vi "Func_ChangeControl.vi"(8 "error in (no error)":errorcluster, 10 "Control Path":path, 11 "Control in":refnum<vi>) -> (0 "error out":errorcluster, 3 "GObject out":refnum<vi>)   [LabVIEW 2010, in "TemplateGenerator.lvlib"]
uses:
  TemplateGenerator.lvlib
  <vilib>/Utility/miscctls.llb/LVPointTypeDef.ctl
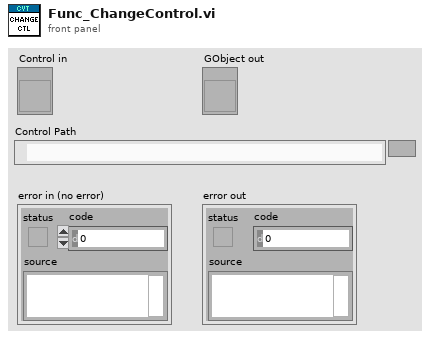
[diagram p1: front panel]
types:
  T1 = typedef "LVPointTypeDef.ctl" = cluster{"Horizontal":i16, "Vertical":i16}
  T2 = typedef "LVNumericRepresentation.ctl" = enum32{"Extended Precision", "Double Precision", "Single Precision", "Long", "Word", "Byte", "Unsigned Long", "Unsigned Word", "Unsigned Byte", "Complex Extended", "Complex Double", "Complex Single", "Quad", "Unsigned Quad", "Fixed-Point"}
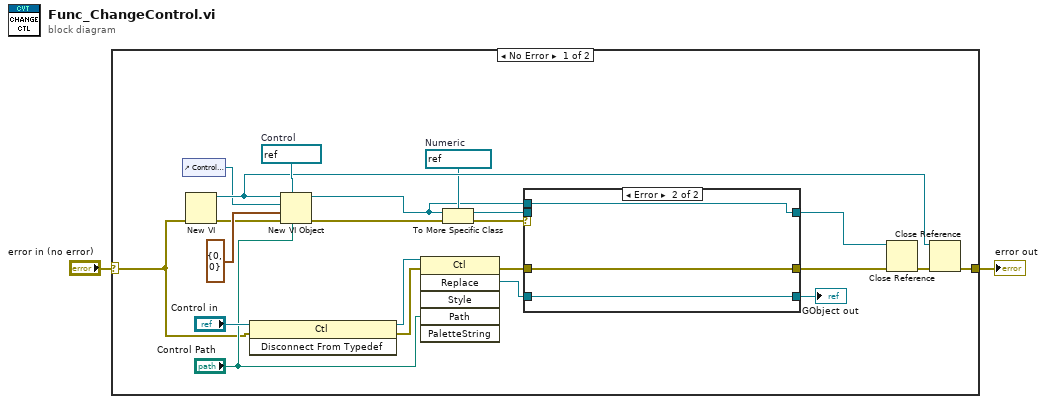
[diagram p0: block diagram]
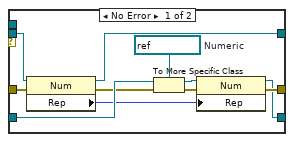
[diagram p2: hidden frame]
diagram:
  n1 = case shown="No Error" "error in (no error)" {
    selector: "error in (no error)" -> [w4 w39]
    tunnel: [w6 w39] -> w2
    frame No Error {
      w17 = refnum<vi> refnum  # Numeric
      w21 = refnum<vi> refnum  # Control
      n2 = control-ref of="Control Path"() -> (w15:refnum<vi>)
      n3 = New VI(8:w4) -> (0:w18:errorcluster, 3:w19:refnum<vi>)  [unwired: 6 in]
      n4 = invoke class="Ctl" method="Disconnect From Typedef"(reference="Control in", error in=w4) -> (reference out=w23:refnum<vi>, error out=w24:errorcluster)  [unwired: 1 in, 1 out]
      n5 = New VI Object(vi object class=w21, owner refnum=w19, style=w15, position/next to=T1 {"Horizontal"=0, "Vertical"=0} ("location"), 6:"Control Path", 8:w18) -> (object refnum=w3:refnum<vi>, 0:w10:errorcluster)  [unwired: 2 in]
      n6 = invoke class="Ctl" method="Replace"(reference=w23, error in=w24, "Path"="Control Path") -> (error out=w5:errorcluster, "Replace"=w13:refnum<vi>)  [unwired: 3 in, 4 out]
      n7 = To More Specific Class(target class=w17, reference=w3, error in=w10) -> (specific class reference=w12:refnum<vi>, error out=w14:errorcluster)
      n8 = case shown="Error" w14 {
        tunnel: w13 -> [w32 w38]
        tunnel: w5 -> [w35 w37]
        tunnel: w12 -> [w34 _]
        tunnel: [w33 w36] -> w11
        tunnel: [w26 w37] -> w8
        tunnel: [w25 w38] -> w9
        tunnel: w3 -> [_ w36]
        frame No Error {
          w31 = refnum<vi> refnum  # Numeric
          n9 = property class="Num"(reference=w34, error in=w35) -> (reference out=w33:refnum<vi>, error out=w29:errorcluster, "Rep"=w27:T2)
          n10 = To More Specific Class(target class=w31, reference=w32, error in=w29) -> (specific class reference=w30:refnum<vi>, error out=w28:errorcluster)
          n11 = property class="Num"(reference=w30, error in=w28, "Rep"=w27) -> (reference out=w25:refnum<vi>, error out=w26:errorcluster)
        }
        frame Error {
        }
      }
      "GObject out" <- w9
      n12 = Close Reference(reference=w11, error in (no error)=w8) -> (error out=w7:errorcluster)
      n13 = Close Reference(reference=w19, error in (no error)=w7) -> (error out=w6:errorcluster)
    }
    frame Error {
    }
  }
  "error out" <- w2
